vi "AlliGator Add New Parameter Map Set.vi"(6 "Parameter Map Names":string[](array[string]), 8 "error in (no error)":errorcluster, 9 "Map Parameter Refnum":refnum<vi>, 10 "New Parameter Map Set":string, 11 "Parameter Map Set Refnum":refnum<vi>) -> (0 "error out":errorcluster, 3 "Build Parameter Map Event Data":T1)   [LabVIEW 2021, in "AlliGator Decay Fit Parameter Map.lvlib"]
uses:
  Decay Fit Parameter Map/AlliGator Decay Fit Parameter Map.lvlib
  AlliGator Parameter Map Update Event Data.ctl
  AlliGator Parameter Map.lvlib
  Strings/Strings.lvlib
panel:
  # "see the License on the block diagram (Ctrl+E or Window:Show Block Diagram)"
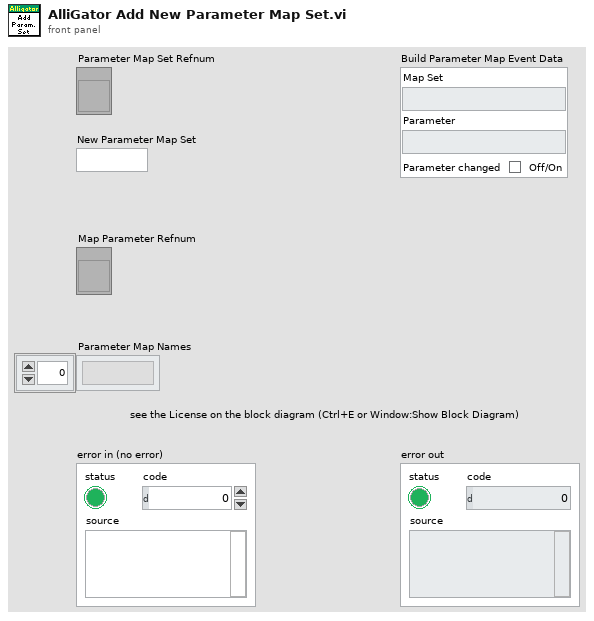
[diagram p1: front panel]
types:
  T1 = typedef "AlliGator Parameter Map.lvlib/AlliGator Parameter Map Update Event Data.ctl" = cluster{"Parameter":u16, "Parameter changed":bool, "Map Set":u16}
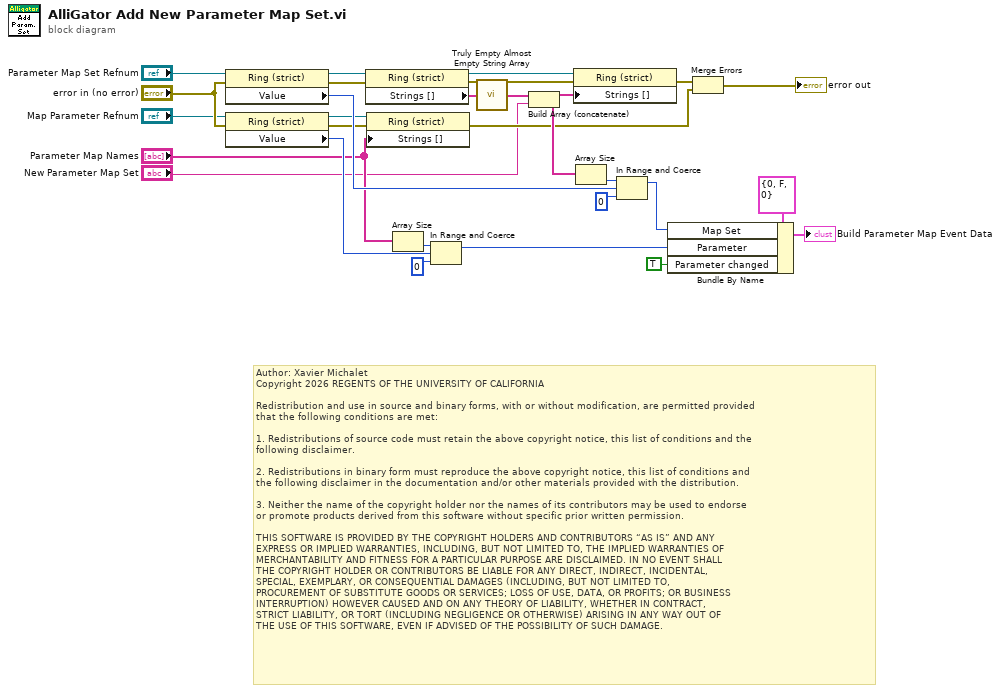
[diagram p0: block diagram]
diagram:
  # "Author: Xavier Michalet\nCopyright 2026 REGENTS OF THE UNIVERSITY OF CALIFORNIA\n\nRedistribution and use in source and binary forms, with or without modification, are permitted provided\nthat the following conditions are met:\n\n1. Redistributions of source code must retain the above copyright notice, this list of conditions and the\nfollowing disclaimer.\n\n2. Redistributions in binary form must reproduce the above copyright notice, this list of conditions and\nthe following disclaimer in the documentation and/or other materials provided with the distribution.\n\n3. Neither the name of the copyright holder nor the names of its contributors may be used to endorse \nor promote products derived from this software without specific prior written permission.\n\nTHIS SOFTWARE IS PROVIDED BY THE COPYRIGHT HOLDERS AND CONTRIBUTORS “AS IS” AND ANY \nEXPRESS OR IMPLIED WARRANTIES, INCLUDING, BUT NOT LIMITED TO, THE IMPLIED WARRANTIES OF\nMERCHANTABILITY AND FITNESS FOR A PARTICULAR PURPOSE ARE DISCLAIMED. IN NO EVENT SHALL\nTHE COPYRIGHT HOLDER OR CONTRIBUTORS BE LIABLE FOR ANY DIRECT, INDIRECT, INCIDENTAL, \nSPECIAL, EXEMPLARY, OR CONSEQUENTIAL DAMAGES (INCLUDING, BUT NOT LIMITED TO, \nPROCUREMENT OF SUBSTITUTE GOODS OR SERVICES; LOSS OF USE, DATA, OR PROFITS; OR BUSINESS\nINTERRUPTION) HOWEVER CAUSED AND ON ANY THEORY OF LIABILITY, WHETHER IN CONTRACT, \nSTRICT LIABILITY, OR TORT (INCLUDING NEGLIGENCE OR OTHERWISE) ARISING IN ANY WAY OUT OF\nTHE USE OF THIS SOFTWARE, EVEN IF ADVISED OF THE POSSIBILITY OF SUCH DAMAGE."
  n1 = property class="Ring (strict)"(reference="Parameter Map Set Refnum", error in="error in (no error)") -> (reference out=w13:refnum<vi>, error out=w14:errorcluster, "Value"=w26:u16)
  n2 = property class="Ring (strict)"(reference="Map Parameter Refnum", error in="error in (no error)") -> (reference out=w15:refnum<vi>, error out=w17:errorcluster, "Value"=w21:u16)
  n3 = property class="Ring (strict)"(reference=w13, error in=w14) -> (reference out=w2:refnum<vi>, error out=w4:errorcluster, "Strings []"=w3:string[])
  n4 = property class="Ring (strict)"(reference=w15, error in=w17, "Strings []"="Parameter Map Names") -> (error out=w9:errorcluster)  [unwired: 1 out]
  n5 = Array Size(array="Parameter Map Names") -> (size(s)=w19:i32)
  n6 = In Range and Coerce(upper limit=w19, x=w21, lower limit=0) -> (coerced(x)=w22:i32)  [unwired: 1 out]
  n7 = call "Truly Empty Almost Empty String Array.vi"("String Array"=w3) -> ("String Array"=w28:string[])  [unwired: 14 in]
  n8 = Build Array (concatenate)(w28, "New Parameter Map Set") -> (w27:string[])
  n9 = property class="Ring (strict)"(reference=w2, error in=w4, "Strings []"=w27) -> (error out=w7:errorcluster)  [unwired: 1 out]
  n10 = Array Size(array=w27) -> (size(s)=w24:i32)
  n11 = In Range and Coerce(upper limit=w24, x=w26, lower limit=0) -> (coerced(x)=w25:i32)  [unwired: 1 out]
  n12 = Bundle By Name(cluster=T1 {"Parameter"=0, "Parameter changed"=FALSE, "Map Set"=0} ("Parameter Map Update Event Data"), "Map Set"=w25, "Parameter"=w22, "Parameter changed"=TRUE) -> (→"Build Parameter Map Event Data":T1)
  n13 = Merge Errors(w7, w9) -> (→"error out":errorcluster)
